vi "BAM Generation Get Next Message.vi"(0 "Connecion Cluster":T2 {"Packets"."Identifier" format="%08x"}, 11 "error in (no error)":errorcluster) -> (4 "Connecion Cluster Out":T2 {"Packets"."Identifier" format="%08x"}, 6 "Data to Send":T1 {"Identifier" format="%08x"}, 8 "Message Available?":bool, 10 "Message Finished?":bool, 15 "error out":errorcluster)   [LabVIEW 2013, in "J1939 Addon Engine.lvlib"]
uses:
  Engine/J1939 Addon Engine.lvlib
  Types/BAM Generation Connection Cluster.ctl
  J1939 Utilities/Types/CAN Outgoing Message Cluster.ctl
  J1939 Utilities/J1939 Utilities.lvlib
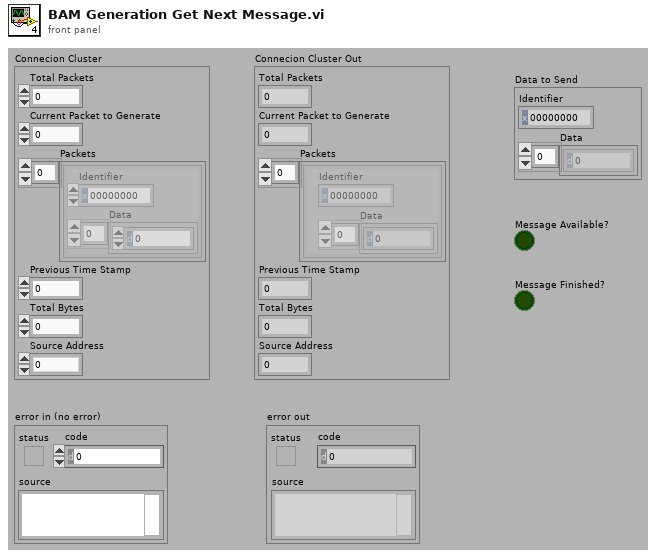
[diagram p1: front panel]
types:
  T1 = typedef "J1939 Addon Shared.lvlib/J1939 Utilities.lvlib/CAN Outgoing Message Cluster.ctl" = cluster{"Identifier":u32, "Data":u8[]}
  T2 = typedef "J1939 Addon Engine.lvlib/BAM Generation Connection Cluster.ctl" = cluster{"Total Packets":u8, "Current Packet to Generate":u8, "Packets":T1[], "Previous Time Stamp":u32, "Total Bytes":u16, "Source Address":u8}
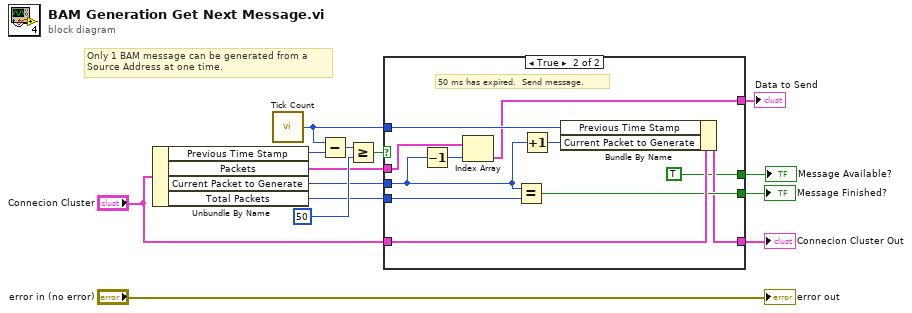
[diagram p0: block diagram]
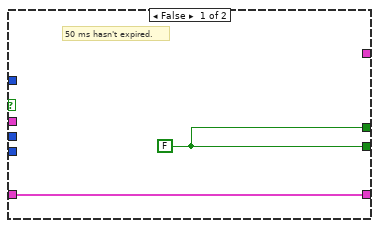
[diagram p2: hidden frame]
diagram:
  # "Only 1 BAM message can be generated from a Source Address at one time."
  n1 = Unbundle By Name("Connecion Cluster") -> ("Previous Time Stamp"=w11:u32, "Packets"=w7:T1[], "Current Packet to Generate"=w6:u8, "Total Packets"=w5:u8)
  n2 = call "Tick Count"() -> ("Tick Count(mSec)"=w1:u32)
  n3 = Subtract(x=w1, y=w11) -> (x-y=w10:u32)
  n4 = Greater Or Equal?(x=w10, y=u32 50) -> (x >= y?=w8:bool)
  n5 = case shown="True" w8 {
    tunnel: w7 -> [_ w24]
    tunnel: w6 -> [_ w22]
    tunnel: w5 -> [_ w17]
    tunnel: "Connecion Cluster" -> [w16 w27]
    tunnel: w1 -> [_ w26]
    tunnel: [_ w23] -> w2
    tunnel: [w15 w21] -> w14
    tunnel: [w16 w20] -> w13
    tunnel: [w15 TRUE ("Message Available?")] -> w3
    frame False {
      w15 = FALSE
      # "50 ms hasn't expired."
    }
    frame True {
      # "50 ms has expired.  Send message."
      n6 = Decrement(x=w22) -> (x-1=w18:u8)
      n7 = Index Array(array=w24, index=w18) -> (element=w23:T1)
      n8 = Equal?(x=w22, y=w17) -> (x = y?=w21:bool)
      n9 = Increment(x=w22) -> (x+1=w25:u8)
      n10 = Bundle By Name(cluster=w27, "Previous Time Stamp"=w26, "Current Packet to Generate"=w25) -> (w20:T2)
    }
  }
  "Message Finished?" <- w14
  "Connecion Cluster Out" <- w13
  "Message Available?" <- w3
  "Data to Send" <- w2
  "error out" <- "error in (no error)"
